vi "GetInterfaceHandle.vi"(3 "error in (no error)":errorcluster, 5 "nIndex":u32) -> (0 "error out":errorcluster, 1 "GX_STATUS":i32, 2 "phIF":u64)   [LabVIEW 2016, in "GxLVLib.lvlib"]
uses:
  GxLVLib.lvlib
  GxIAPI.dll
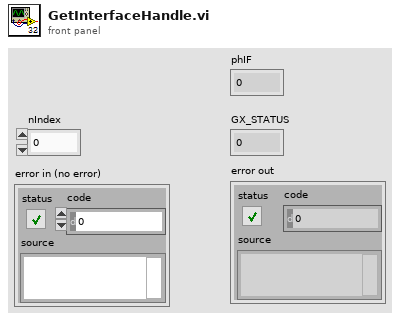
[diagram p1: front panel]
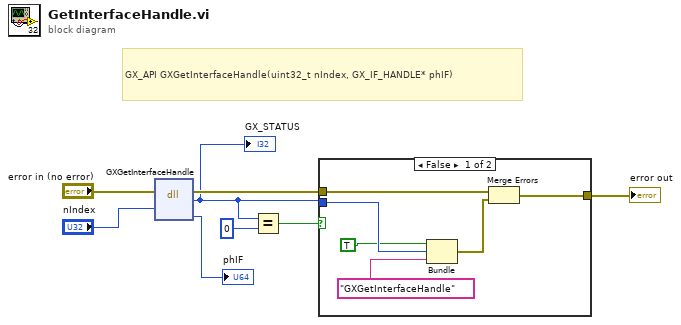
[diagram p0: block diagram]
diagram:
  # "GX_API GXGetInterfaceHandle(uint32_t nIndex, GX_IF_HANDLE* phIF)"
  n1 = dll-call lib="GxIAPI.dll" fn="GXGetInterfaceHandle"(error in="error in (no error)", "nIndex"="nIndex") -> (error out=w5:errorcluster, "GX_STATUS"=w1:i32, "phIF"=→"phIF":i64)  [unwired: 4 in, 1 out]
  "GX_STATUS" <- w1
  n2 = Equal?(x=w1, y=0) -> (x = y?=w3:bool)
  n3 = case shown="False" w3 {
    tunnel: w5 -> [w14 w15]
    tunnel: [w13 w15] -> w6
    tunnel: w1 -> [w10 _]
    frame False {
      n4 = Bundle(TRUE, "GX_STATUS"=w10, "GXGetInterfaceHandle") -> (w11:cluster{bool, "GX_STATUS":i32, string})  [unwired: 1 in]
      n5 = Merge Errors(w14, w11) -> (w13:errorcluster)
    }
    frame True {
    }
  }
  "error out" <- w6
